vi "Motion Profile Generater-Optimized.vi"(0 "Max Speed (rotations/sec)":dbl, 5 "Max Acceleration (rotations/sec^2)":dbl, 7 "Max Jerk (rotations/sec^3)":dbl, 9 "Rotations to Travel":dbl, 11 "Motion Profile Control Frame Rate":dbl) -> (4 "Position rotations":dbl[](array[numeric]), 6 "velocity rotations/sec":dbl[](array[numeric]))   [LabVIEW 2015]
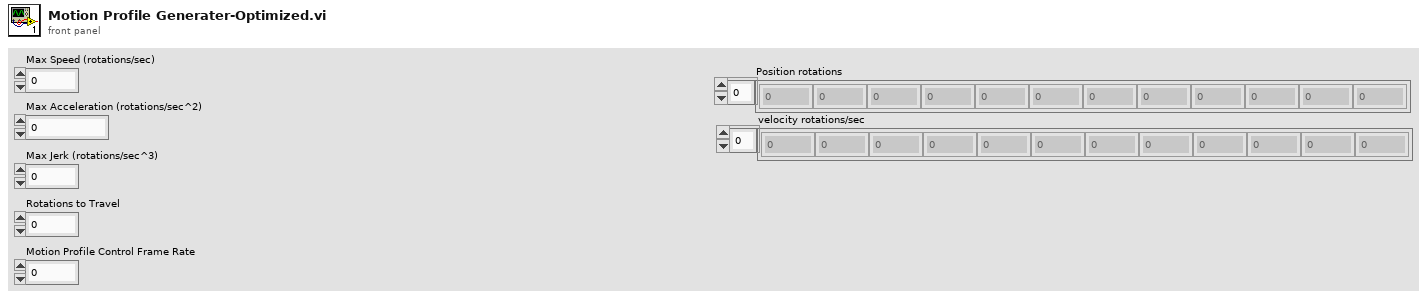
[diagram p1: front panel]
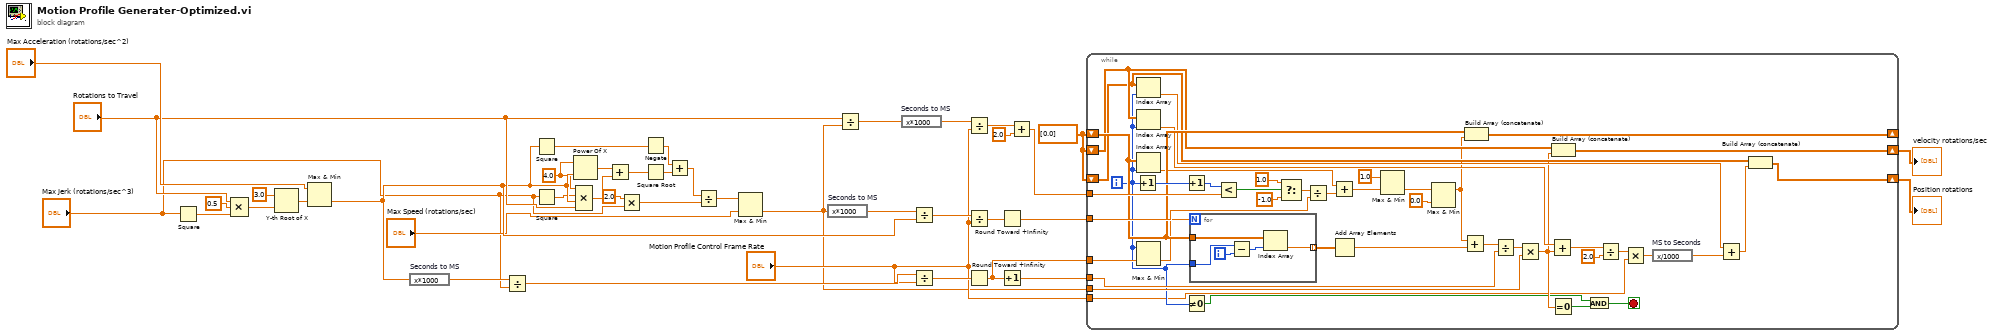
[diagram p0: block diagram]
diagram:
  w9 = 4.0 ("x")
  w18 = dbl[] [0.0]
  n1 = Square(x="Max Jerk (rotations/sec^3)") -> (x^2=w15:dbl)
  n2 = Compound Arithmetic op=MULTIPLY("Rotations to Travel", 0.5 ("value"), w15) -> (w14:dbl)
  n3 = Y-th Root of X(1:w14, 2:3.0 ("y")) -> (0:w17:dbl)
  n4 = Max & Min(x="Max Acceleration (rotations/sec^2)", y=w17) -> (min(x,y)=w22:dbl)  [unwired: 1 out]
  n5 = expression code="x*1000" "Seconds to MS"(w22) -> (w41:dbl)
  n6 = Divide(x=w41, y="Max Jerk (rotations/sec^3)") -> (x/y=w31:dbl)
  n7 = Square(x=w22) -> (x^2=w12:dbl)
  n8 = Square(x="Max Jerk (rotations/sec^3)") -> (x^2=w8:dbl)
  n9 = Power Of X(1:w22, 2:w9) -> (0:w10:dbl)
  n10 = Compound Arithmetic op=MULTIPLY(w9, w8, w22, "Rotations to Travel") -> (w7:dbl)
  n11 = Add(x=w10, y=w7) -> (x+y=w6:dbl)
  n12 = Multiply(x=2.0, y="Max Jerk (rotations/sec^3)") -> (x*y=w1:dbl)
  n13 = Negate(x=w12) -> (-x=w11:dbl)
  n14 = Square Root(x=w6) -> (sqrt(x)=w4:dbl)
  n15 = Add(x=w11, y=w4) -> (x+y=w3:dbl)
  n16 = Divide(x=w3, y=w1) -> (x/y=w2:dbl)
  n17 = Max & Min(x=w2, y="Max Speed (rotations/sec)") -> (min(x,y)=w20:dbl)  [unwired: 1 out]
  n18 = expression code="x*1000" "Seconds to MS"(w20) -> (w40:dbl)
  n19 = Divide(x="Rotations to Travel", y=w20) -> (x/y=w39:dbl)
  n20 = expression code="x*1000" "Seconds to MS"(w39) -> (w38:dbl)
  n21 = Divide(x=w40, y=w22) -> (x/y=w34:dbl)
  n22 = Divide(x=w31, y="Motion Profile Control Frame Rate") -> (x/y=w30:dbl)
  n23 = Divide(x=w38, y="Motion Profile Control Frame Rate") -> (x/y=w37:dbl)
  n24 = Divide(x=w34, y="Motion Profile Control Frame Rate") -> (x/y=w33:dbl)
  n25 = Round Toward +Infinity(x=w30) -> (ceil(x): smallest int >= x=w29:dbl)
  n26 = Round Toward +Infinity(x=w33) -> (ceil(x): smallest int >= x=w32:dbl)
  n27 = Increment(x=w29) -> (x+1=w28:dbl)
  n28 = Add(x=w37, y=2.0) -> (x+y=w35:dbl)
  n29 = while {
    tunnel: w35 -> [w84]
    shift-right: [w71] -> _
    shift-left: w18 -> [w70]
    tunnel: w32 -> [w76]
    tunnel: w29 -> [w68]
    tunnel: w28 -> [w64]
    tunnel: w20 -> [w62]
    shift-right: [w61] -> w26
    shift-left: w18 -> [w59]
    shift-right: [w60] -> w25
    shift-left: w18 -> [w53]
    tunnel: "Motion Profile Control Frame Rate" -> [w42]
    i -> [w43]
    stop <- w46 stop-if-true
    n30 = Increment(x=w43) -> (x+1=w73:i32)
    n31 = Index Array(array=w53, index=w43) -> (element=w52:dbl)
    n32 = Index Array(array=w59, index=w43) -> (element=w50:dbl)
    n33 = Index Array(array=w70, index=w43) -> (element=w44:dbl)
    n34 = Max & Min(x=w43, y=w68) -> (min(x,y)=w67:dbl)  [unwired: 1 out]
    n35 = Increment(x=w73) -> (x+1=w74:i32)
    n36 = Not Equal To 0?(x=w43) -> (x != 0?=w47:bool)
    n37 = for {
      N: w67 -> [_]
      tunnel: w43 -> [w88]
      tunnel: w70 -> [w86]
      tunnel: [w85] -> w69 mode=indexing
      i -> [w89]
      n38 = Subtract(x=w88, y=w89) -> (x-y=w87:i32)
      n39 = Index Array(array=w86, index=w87) -> (element=w85:dbl)
    }
    n40 = Less?(x=w74, y=w84) -> (x < y?=w80:bool)
    n41 = Select(t=1.0, s=w80, f=-1.0) -> (s? t:f=w77:dbl)
    n42 = Divide(x=w77, y=w76) -> (x/y=w75:dbl)
    n43 = Add(x=w44, y=w75) -> (x+y=w72:dbl)
    n44 = Add Array Elements(numeric array=w69) -> (sum=w66:dbl)
    n45 = Max & Min(x=1.0, y=w72) -> (min(x,y)=w82:dbl)  [unwired: 1 out]
    n46 = Max & Min(x=w82, y=0.0) -> (max(x,y)=w45:dbl)  [unwired: 1 out]
    n47 = Add(x=w45, y=w66) -> (x+y=w65:dbl)
    n48 = Build Array (concatenate)(w70, w45) -> (w71:dbl[])
    n49 = Divide(x=w65, y=w64) -> (x/y=w63:dbl)
    n50 = Multiply(x=w63, y=w62) -> (x*y=w49:dbl)
    n51 = Add(x=w50, y=w49) -> (x+y=w58:dbl)
    n52 = Equal To 0?(x=w49) -> (x = 0?=w48:bool)
    n53 = Build Array (concatenate)(w59, w49) -> (w61:dbl[])
    n54 = And(x=w47, y=w48) -> (x .and. y?=w46:bool)
    n55 = Divide(x=w58, y=2.0) -> (x/y=w56:dbl)
    n56 = Multiply(x=w56, y=w42) -> (x*y=w55:dbl)
    n57 = expression code="x/1000" "MS to Seconds"(w55) -> (w54:dbl)
    n58 = Add(x=w52, y=w54) -> (x+y=w51:dbl)
    n59 = Build Array (concatenate)(w53, w51) -> (w60:dbl[])
  }
  "velocity rotations/sec" <- w26
  "Position rotations" <- w25
